vi "dialogue.vi"(0 "Cancel":bool, 1 "OK":bool, 2 "Author":string, 10 "HDF5 Save":path[](array[path])=[path "", path ""], 11 "RID":string) -> ()   [LabVIEW 2013]
uses:
  <vilib>/addons/h5labview2/file/H5Fmode.ctl
  <vilib>/addons/h5labview2/base/lib_path.vi
  <vilib>/addons/h5labview2/base/H5Equery.vi
  <vilib>/addons/h5labview2/attrib/H5Awrite.llb/H5Awrite.xnode
  <vilib>/addons/h5labview2/file/H5F.lvlib
panel:
  in  "Description":string
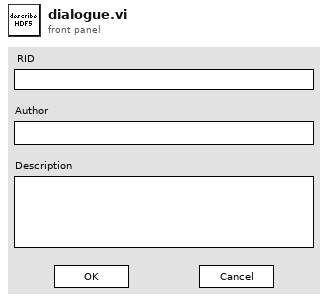
[diagram p1: front panel]
types:
  T1 = typedef "H5F.lvlib/H5Fmode.ctl" = enum16{"read-only", "read-write", "overwrite", "create new", "open or create"}
  T2 = typedef "Semaphore RefNum" = refnum<k1>
  T3 = typedef "hid_t.ctl" = i32
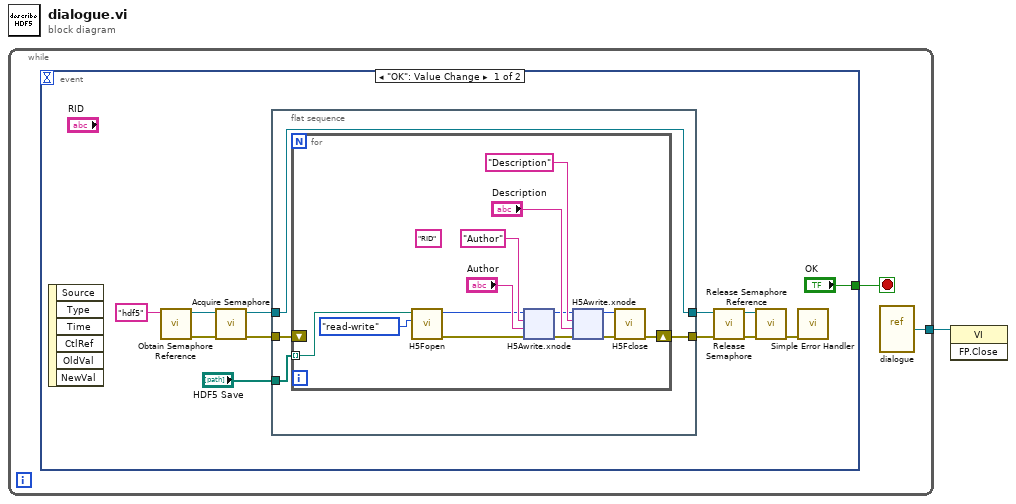
[diagram p0: block diagram]
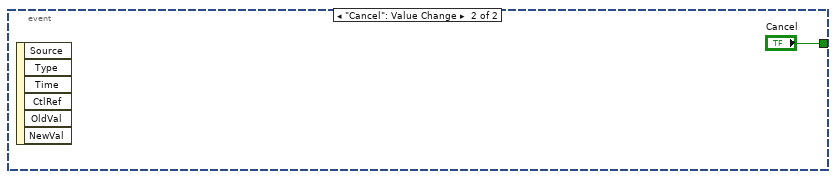
[diagram p2: hidden frame]
diagram:
  n1 = while {
    tunnel: [w2] -> w1
    stop <- w3 stop-if-true
    n2 = event shown="[0] \"OK\": Value Change" {
      selector: _ -> [_ _]
      dyn-events: _ -> [_ _]
      timeout: _ -> [_ _]
      tunnel: ["OK" "Cancel"] -> w3
      event "OK": Value Change {
        n3 = event-data() -> ()  [unwired: 1 in, 6 out]
        n4 = call <vilib>:"Obtain Semaphore Reference.vi"("name (unnamed)"="hdf5") -> ("error out"=w13:errorcluster, "semaphore"=w14:T2)  [unwired: 4 in, 1 out]
        n5 = call <vilib>:"Acquire Semaphore.vi"("error in (no error)"=w13, "semaphore"=w14) -> ("error out"=w7:errorcluster, "semaphore out"=w8:T2)  [unwired: 3 in, 1 out]
        n6 = flat-sequence {
          tunnel: [w19] -> w9
          tunnel: w8 -> [w19]
          tunnel: w7 -> [w17]
          tunnel: "HDF5 Save" -> [w18]
          tunnel: [w16] -> w5
          frame #0 {
            n7 = for {
              tunnel: w18 -> [w31] mode=indexing
              shift-right: [w22] -> w16
              shift-left: w17 -> [_]
              (unwired) "RID" ("attrib name")
              n8 = call <vilib>:"H5Fopen.vi"("mode (read-only)"=H5Fmode."read-write", "path"=w31) -> ("error out"=w20:errorcluster, "ref out"=w21:T3)  [unwired: 8 in]
              n9 = xnode "H5Awrite.xnode"("error in (no error)"=w20, "data"="Author", "attrib name"="Author", "ref in"=w21) -> ("error out"=w28:errorcluster, "ref out"=w25:i32)  [unwired: 3 in, 1 out]
              n10 = xnode "H5Awrite.xnode"("error in (no error)"=w28, "data"="Description", "attrib name"="Description", "ref in"=w25) -> ("error out"=w24:errorcluster, "ref out"=w23:i32)  [unwired: 3 in, 1 out]
              n11 = call <vilib>:"H5Fclose.vi"("error in (no error)"=w24, "ref"=w23) -> ("error out"=w22:errorcluster)  [unwired: 9 in]
            }
          }
        }
        n12 = call <vilib>:"Release Semaphore.vi"("error in (no error)"=w5, "semaphore"=w9) -> ("error out"=w11:errorcluster, "semaphore out"=w10:T2)  [unwired: 4 in]
        n13 = call <vilib>:"Release Semaphore Reference.vi"("error in (no error)"=w11, "semaphore"=w10) -> ("error out"=w4:errorcluster)  [unwired: 8 in, 1 out]
        n14 = call <vilib>:"Simple Error Handler.vi"("error in (no error)"=w4) -> ()  [unwired: 4 in, 5 out]
      }
      event "Cancel": Value Change {
        n15 = event-data() -> ()  [unwired: 1 in, 6 out]
      }
    }
    n16 = vi-ref "dialogue.vi"() -> (w2:refnum<vi>)
  }
  n17 = invoke class="VI" method="FP.Close"(reference=w1) -> ()  [unwired: 2 in, 3 out]
